vi "0x2 RIO-OCU update send.vi"(11 "OCU Writer In":refnum<class "NetworkStreamWriter.lvclass">) -> (3 "OCU Writer Out":refnum<class "NetworkStreamWriter.lvclass">)   [LabVIEW 2011]
doc: "Sends general data up to the listening OCU over a network stream for monitoring and debugging purposes."
uses:
  0x2 Classes/NetworkStreams/Writer/NetworkStreamWriter.lvclass
  0x2 Typedefs/RIO-OCU update controls.ctl
  2-Think/2 Typedefs/generalized sensor status.ctl
  2-Think/2 Typedefs/indicator LED.ctl
  2-Think/2 Typedefs/generalized actuator status.ctl
  2-Think/2 Typedefs/Which Boat.ctl
  2-Think/2 Typedefs/robot velocity.ctl
  2-Think/2 Typedefs/UTM Location.ctl
  2-Think/2 Typedefs/heading.ctl
  2-Think/2 Typedefs/rate of turn.ctl
  2-Think/2 Typedefs/pitch and roll.ctl
  2-Think/2 Typedefs/apparent wind.ctl
  2-Think/2 Typedefs/apparent wind speed.ctl
  2-Think/2 Typedefs/apparent wind direction.ctl
  2-Think/2 Typedefs/Velocity.ctl
  2-Think/2 Typedefs/absolute wind direction.ctl
  2-Think/2 Typedefs/absolute wind speed.ctl
  2-Think/2 Typedefs/absolute water current vector.ctl
  2-Think/2 Typedefs/rudder angle.ctl
  2-Think/2 Typedefs/sail setpt.ctl
  0x2 Typedefs/manual override.ctl
  2-Think/2 Typedefs/setpoints to boat.ctl
  0x2 Typedefs/Current Waypoint.ctl
  2-Think/2 Typedefs/Goodness Fns Indicator.ctl
  2-Think/2 Typedefs/UTM Circle.ctl
  2-Think/2 Globals/2 Global.vi
  2-Think/2 Classes/MissionQueue/MissionQueue.lvclass
panel:
  out "output cluster":T1 {"Absolute Wind"."East" format="%#_5g"; "Robot Pitch/Roll"."Roll" format="%05.1f"; "Robot Pitch/Roll"."Pitch" format="%05.1f"; "Robot\nRate of Turn" format="%05.1f"; "Robot\nHeading" format="%05.1f"; "Robot UTM Location"."North" format="%#_10f"; "Robot UTM Location"."East" format="%#_8f"}
  # "How Am I?"
  # "Where Am I?"
  # "Path Planning"
  # "From Planning Functions"
  # "(this is not a cluster because subitems\nare generated in parallel code)"
  # "What's Around Me?"
  # "As Measured"
  # "As Measured"
  # "Loop Rates"
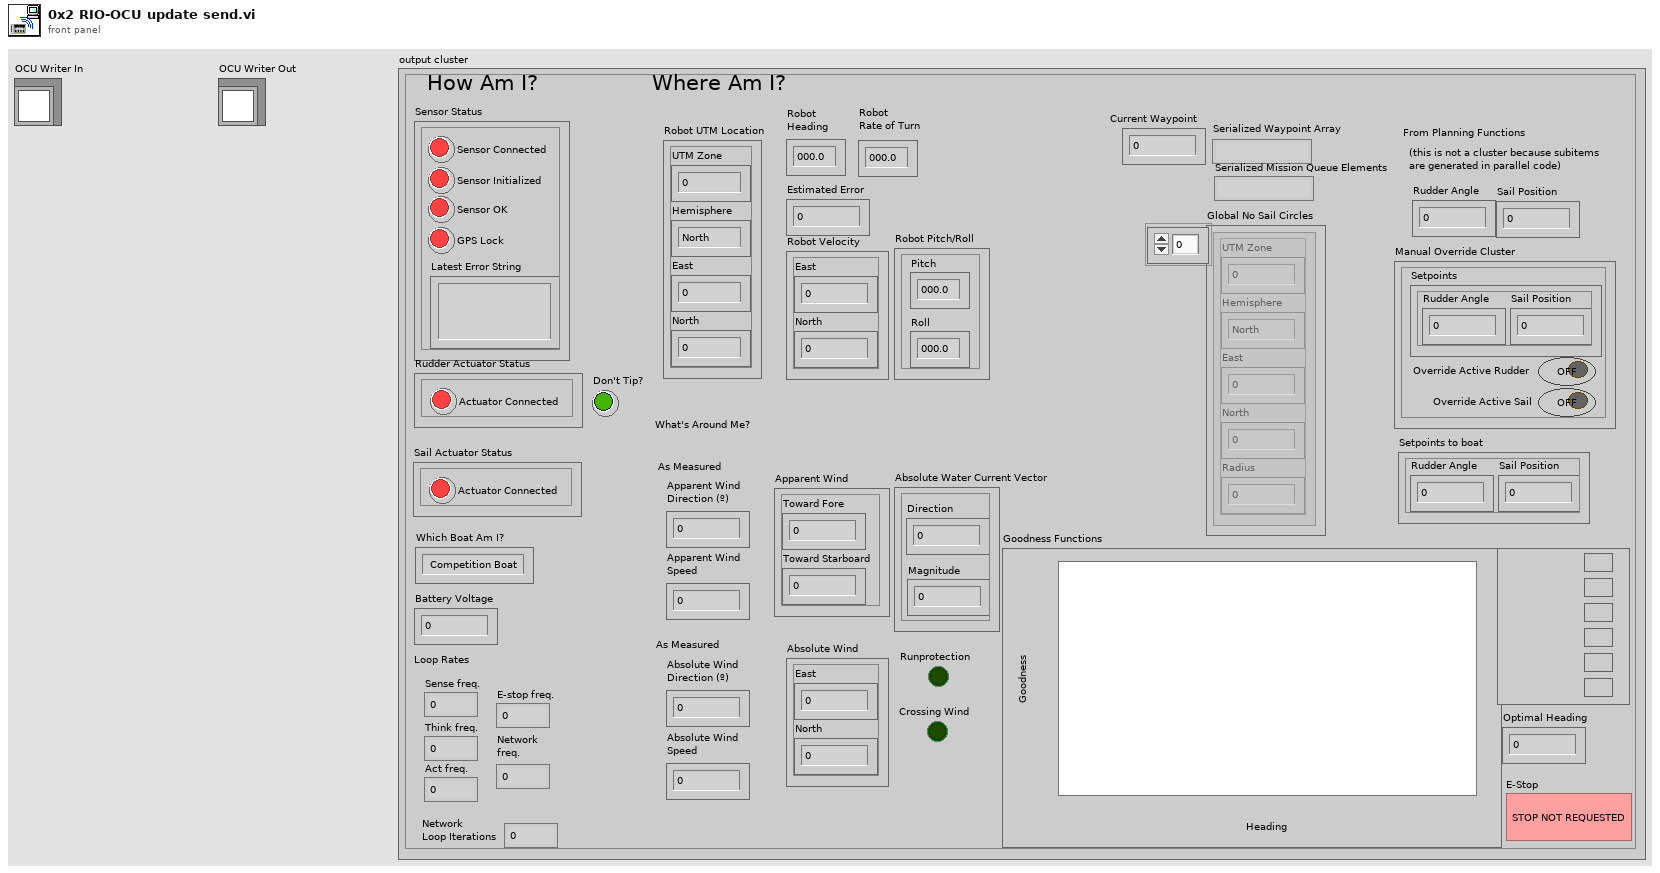
[diagram p1: front panel]
types:
  T1 = typedef "RIO-OCU update controls.ctl" = cluster{"Sensor Status":T2, "Battery Voltage":dbl, "Rudder Actuator Status":T4, "Sail Actuator Status":T4, "Which Boat Am I?":T5, "Robot Velocity":T6, "Robot UTM Location":T7, "Robot\nHeading ":T8, "Robot\nRate of Turn":T9, "Robot Pitch/Roll":T10, "Apparent Wind":T11, "Apparent Wind\nSpeed":T12, "Apparent Wind\nDirection (º)":T13, "Absolute Wind":T14, "Absolute Wind\nDirection (º)":T15, "Absolute Wind\nSpeed":T16, "Absolute Water Current Vector":T17, "Rudder Angle":T18, "Sail Position":T19, "Manual Override Cluster":T20, "Setpoints to boat":T21, "Current Waypoint":T22, "Think freq.":dbl, "Sense freq.":dbl, "Act freq.":dbl, "E-stop freq.":dbl, "Network \nfreq.":dbl, "Network \nLoop Iterations":i64, "E-Stop":bool, "Serialized Waypoint Array":string, "Serialized Mission Queue Elements":string, "Goodness Functions":T23, "Global No Sail Circles":T24[], "Runprotection":bool, "Optimal Heading":dbl, "Crossing Wind":bool, "Estimated Error":dbl, "Don't Tip?":bool}
  T2 = typedef "generalized sensor status.ctl" = cluster{"Sensor Connected":T3, "Sensor Initialized":T3, "Sensor OK":T3, "Latest Error String":string, "GPS Lock":T3}
  T3 = typedef "indicator LED.ctl" = bool
  T4 = typedef "generalized actuator status.ctl" = cluster{"Actuator Connected":T3}
  T5 = typedef "Which Boat.ctl" = enum16{"Competition Boat", "Small RC", "Simulation"}
  T6 = typedef "robot velocity.ctl" = cluster{"East":dbl, "North":dbl}
  T7 = typedef "UTM Location.ctl" = cluster{"UTM Zone":dbl, "Hemisphere":enum16{"North", "South"}, "East":dbl, "North":dbl}
  T8 = typedef "heading.ctl" = dbl
  T9 = typedef "rate of turn.ctl" = dbl
  T10 = typedef "pitch and roll.ctl" = cluster{"Pitch":dbl, "Roll":dbl}
  T11 = typedef "apparent wind.ctl" = cluster{"Toward Fore":dbl, "Toward Starboard":dbl}
  T12 = typedef "apparent wind speed.ctl" = dbl
  T13 = typedef "apparent wind direction.ctl" = dbl
  T14 = typedef "Velocity.ctl" = cluster{"East":dbl, "North":dbl}
  T15 = typedef "absolute wind direction.ctl" = dbl
  T16 = typedef "absolute wind speed.ctl" = dbl
  T17 = typedef "absolute water current vector.ctl" = cluster{"Direction":T13, "Magnitude":T13}
  T18 = typedef "rudder angle.ctl" = dbl
  T19 = typedef "sail setpt.ctl" = dbl
  T20 = typedef "manual override.ctl" = cluster{"Override Active Rudder":bool, "Setpoints":T21, "Override Active Sail":bool}
  T21 = typedef "setpoints to boat.ctl" = cluster{"Sail Position":T19, "Rudder Angle":T18}
  T22 = typedef "Current Waypoint.ctl" = i32
  T23 = typedef "Goodness Fns Indicator.ctl" = cluster{dbl, dbl, dbl[][]}
  T24 = typedef "UTM Circle.ctl" = cluster{"UTM Zone":dbl, "Hemisphere":enum16{"North", "South"}, "East":dbl, "North":dbl, "Radius":dbl}
  T25 = typedef "Waypoints List.ctl" = refnum<class "Waypoint.lvclass">[]
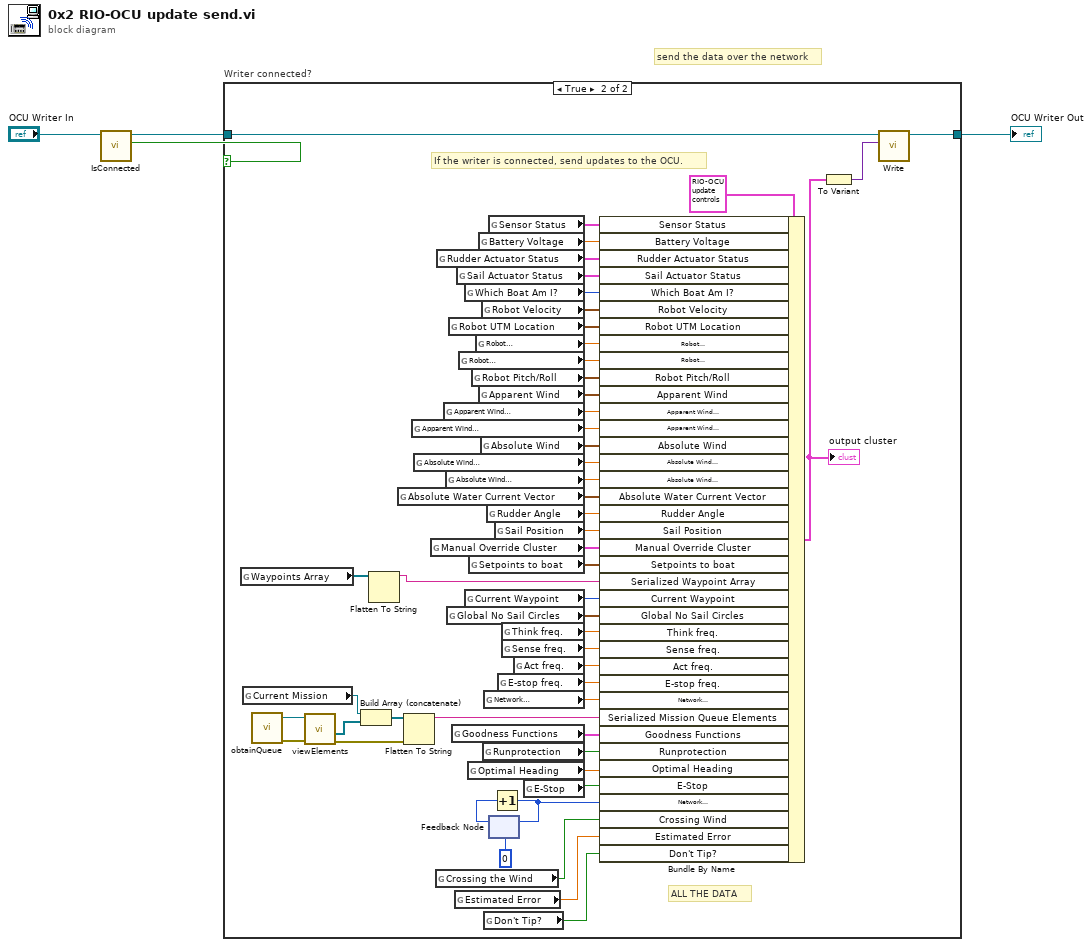
[diagram p0: block diagram]
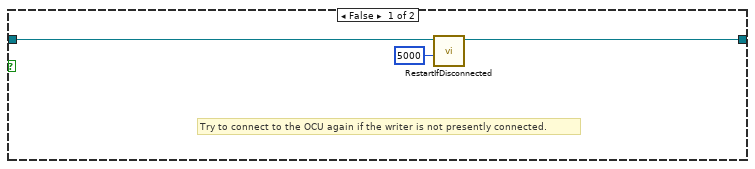
[diagram p2: hidden frame]
diagram:
  # "send the data over the network"
  n1 = call "IsConnected.vi"("NetworkStreamWriter in"="OCU Writer In") -> ("Connected?"=w3:bool, "NetworkStreamWriter out"=w2:refnum<class "NetworkStreamWriter.lvclass">)  [unwired: 8 in, 1 out]
  n2 = case "Writer connected?" shown="True" w3 {
    tunnel: w2 -> [w7 w28]
    tunnel: [w6 w25] -> w1
    frame False {
      # "Try to connect to the OCU again if the writer is not presently connected."
      n3 = call "RestartIfDisconnected.vi"("connection timeout"=5000, "NetworkStreamWriter in"=w7) -> ("NetworkStreamWriter out"=w6:refnum<class "NetworkStreamWriter.lvclass">)  [unwired: 8 in, 1 out]
    }
    frame True {
      # "If the writer is connected, send updates to the OCU."
      # "ALL THE DATA"
      n4 = global read "2 Global.vi" "Waypoints Array"() -> (w19:T25)
      n5 = global read "2 Global.vi" "Current Mission"() -> (w11:refnum<class "GenericMission.lvclass">)
      n6 = call "obtainQueue.vi"() -> ("Error Out"=w23:errorcluster, "MissionQueue.lvclass"=w24:refnum<class "MissionQueue.lvclass">)  [unwired: 10 in]
      n7 = call "viewElements.vi"("error in (no error)"=w23, "MissionQueue in"=w24) -> ("error out"=w22:errorcluster, "elements"=w13:refnum<class "GenericMission.lvclass">[])  [unwired: 5 in, 2 out]
      n8 = Build Array (concatenate)(w11, w13) -> (w12:refnum<class "GenericMission.lvclass">[])
      n9 = Flatten To String(anything=w19) -> (data string=w20:string)  [unwired: 3 in, 2 out]
      n10 = global read "2 Global.vi" "Absolute Water Current Vector"() -> (w56:T14)
      n11 = Flatten To String(anything=w12, error in (no error)=w22) -> (data string=w21:string)  [unwired: 2 in, 2 out]
      n12 = global read "2 Global.vi" "Apparent Wind\nDirection (º)"() -> (w42:T13)
      n13 = global read "2 Global.vi" "Absolute Wind\nDirection (º)"() -> (w43:T15)
      n14 = global read "2 Global.vi" "Manual Override Cluster"() -> (w37:T20)
      n15 = global read "2 Global.vi" "Crossing the Wind"() -> (w10:bool)
      n16 = global read "2 Global.vi" "Rudder Actuator Status"() -> (w49:T4)
      n17 = global read "2 Global.vi" "Apparent Wind\nSpeed"() -> (w41:T12)
      n18 = global read "2 Global.vi" "Absolute Wind\nSpeed"() -> (w44:T16)
      n19 = global read "2 Global.vi" "Global No Sail Circles"() -> (w17:T24[])
      n20 = global read "2 Global.vi" "Robot UTM Location"() -> (w52:T7)
      n21 = global read "2 Global.vi" "Goodness Functions"() -> (w18:T23)
      n22 = global read "2 Global.vi" "Estimated Error"() -> (w9:dbl)
      n23 = global read "2 Global.vi" "Sail Actuator Status"() -> (w50:T4)
      n24 = global read "2 Global.vi" "Robot\nRate of Turn"() -> (w45:T9)
      n25 = global read "2 Global.vi" "Which Boat Am I?"() -> (w47:T5)
      n26 = global read "2 Global.vi" "Current Waypoint"() -> (w38:T22)
      n27 = global read "2 Global.vi" "Optimal Heading"() -> (w14:dbl)
      n28 = global read "2 Global.vi" "Setpoints to boat"() -> (w39:T21)
      n29 = global read "2 Global.vi" "Robot Pitch/Roll"() -> (w53:T10)
      n30 = global read "2 Global.vi" "Robot\nHeading"() -> (w46:T8)
      n31 = global read "2 Global.vi" "Battery Voltage"() -> (w36:dbl)
      n32 = global read "2 Global.vi" "Apparent Wind"() -> (w54:T11)
      n33 = global read "2 Global.vi" "Absolute Wind"() -> (w55:T14)
      n34 = global read "2 Global.vi" "Robot Velocity"() -> (w51:T6)
      n35 = global read "2 Global.vi" "Runprotection"() -> (w16:bool)
      n36 = global read "2 Global.vi" "Network \nfreq."() -> (w34:dbl)
      n37 = global read "2 Global.vi" "Don't Tip?"() -> (w8:bool)
      n38 = global read "2 Global.vi" "Rudder Angle"() -> (w40:T18)
      n39 = global read "2 Global.vi" "Sensor Status"() -> (w48:T2)
      n40 = feedback #1(i64 0) -> (w58:i64)
      n41 = Increment(x=w58) -> (x+1=w59:i64)
      n42 = feedback-in #1(w59) -> ()
      n43 = global read "2 Global.vi" "Sail Position"() -> (w35:T19)
      n44 = global read "2 Global.vi" "E-stop freq."() -> (w33:dbl)
      n45 = global read "2 Global.vi" "Think freq."() -> (w30:dbl)
      n46 = global read "2 Global.vi" "Sense freq."() -> (w31:dbl)
      n47 = global read "2 Global.vi" "Act freq."() -> (w32:dbl)
      n48 = global read "2 Global.vi" "E-Stop"() -> (w15:bool)
      n49 = Bundle By Name(cluster=T1 {"Sensor Status"={"Sensor Connected"=FALSE, "Sensor Initialized"=FALSE, "Sensor OK"=FALSE, "Latest Error String"="", "GPS Lock"=FALSE}, "Battery Voltage"=0.0, "Rudder Actuator Status"={"Actuator Connected"=FALSE}, "Sail Actuator Status"={"Actuator Connected"=FALSE}, "Which Boat Am I?"=enum."Competition Boat", "Robot Velocity"={"East"=0.0, "North"=0.0}, "Robot UTM Location"={"UTM Zone"=0.0, "Hemisphere"=enum."North", "East"=0.0, "North"=0.0}, "Robot\nHeading "=0.0, "Robot\nRate of Turn"=0.0, "Robot Pitch/Roll"={"Pitch"=0.0, "Roll"=0.0}, "Apparent Wind"={"Toward Fore"=0.0, "Toward Starboard"=0.0}, "Apparent Wind\nSpeed"=0.0, "Apparent Wind\nDirection (º)"=0.0, "Absolute Wind"={"East"=0.0, "North"=0.0}, "Absolute Wind\nDirection (º)"=0.0, "Absolute Wind\nSpeed"=0.0, "Absolute Water Current Vector"={"Direction"=0.0, "Magnitude"=0.0}, "Rudder Angle"=0.0, "Sail Position"=0.0, "Manual Override Cluster"={"Override Active Rudder"=FALSE, "Setpoints"={"Sail Position"=0.0, "Rudder Angle"=0.0}, "Override Active Sail"=FALSE}, "Setpoints to boat"={"Sail Position"=0.0, "Rudder Angle"=0.0}, "Current Waypoint"=0, "Think freq."=0.0, "Sense freq."=0.0, "Act freq."=0.0, "E-stop freq."=0.0, "Network \nfreq."=0.0, "Network \nLoop Iterations"=0, "E-Stop"=FALSE, "Serialized Waypoint Array"="", "Serialized Mission Queue Elements"="", "Goodness Functions"={0.0, 0.0, []}, "Global No Sail Circles"=[], "Runprotection"=FALSE, "Optimal Heading"=0.0, "Crossing Wind"=FALSE, "Estimated Error"=0.0, "Don't Tip?"=FALSE} ("Monitored Items from RIO"), "Sensor Status"=w48, "Battery Voltage"=w36, "Rudder Actuator Status"=w49, "Sail Actuator Status"=w50, "Which Boat Am I?"=w47, "Robot Velocity"=w51, "Robot UTM Location"=w52, "Robot\nHeading"=w46, "Robot\nRate of Turn"=w45, "Robot Pitch/Roll"=w53, "Apparent Wind"=w54, "Apparent Wind\nSpeed"=w41, "Apparent Wind\nDirection (º)"=w42, "Absolute Wind"=w55, "Absolute Wind\nDirection (º)"=w43, "Absolute Wind\nSpeed"=w44, "Absolute Water Current Vector"=w56, "Rudder Angle"=w40, "Sail Position"=w35, "Manual Override Cluster"=w37, "Setpoints to boat"=w39, "Serialized Waypoint Array"=w20, "Current Waypoint"=w38, "Global No Sail Circles"=w17, "Think freq."=w30, "Sense freq."=w31, "Act freq."=w32, "E-stop freq."=w33, "Network \nfreq."=w34, "Serialized Mission Queue Elements"=w21, "Goodness Functions"=w18, "Runprotection"=w16, "Optimal Heading"=w14, "E-Stop"=w15, "Network \nLoop Iterations"=w59, "Crossing Wind"=w10, "Estimated Error"=w9, "Don't Tip?"=w8) -> (w27:T1)
      "output cluster" <- w27
      n50 = To Variant(anything=w27) -> (Variant=w26:variant)
      n51 = call "Write.vi"("element"=w26, "NetworkStreamWriter in"=w28) -> ("NetworkStreamWriter out"=w25:refnum<class "NetworkStreamWriter.lvclass">)  [unwired: 7 in, 2 out]
    }
  }
  "OCU Writer Out" <- w1
